vi "Response Check.vi"(6 "Source (\"\")":string, 8 "error in (no error)":errorcluster, 9 "Message In (\"\")":string, 11 "VISA resource name":refnum<visa-resource-name>) -> (0 "error out":errorcluster, 1 "Internal Error Number":i32 max=999 step=1, 2 "Response Type":i32(ring) items=["Affirmative", "Single Negative", "Multiple Negative", "ASCII", "Binary", "End"], 3 "VISA resource name out":refnum<visa-resource-name>, 4 "Internal Error String":string)   [LabVIEW 2020, in "Yokogawa GX Series.lvlib"]
doc: "This VI checks the message.\nThen this returns Internal Error Type.\nIf the message is an error message, this sets \"command are not processed succesfully\" to error out."
uses:
  <instrlib>/Yokogawa GX Series/Yokogawa GX Series.lvlib
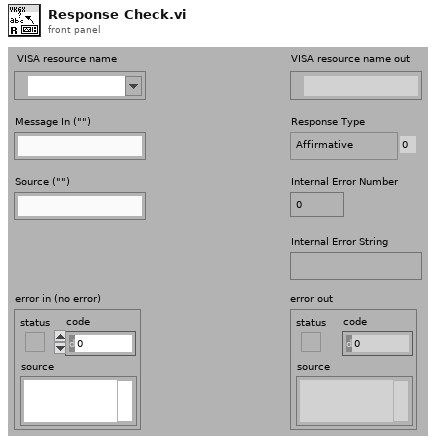
[diagram p1: front panel]
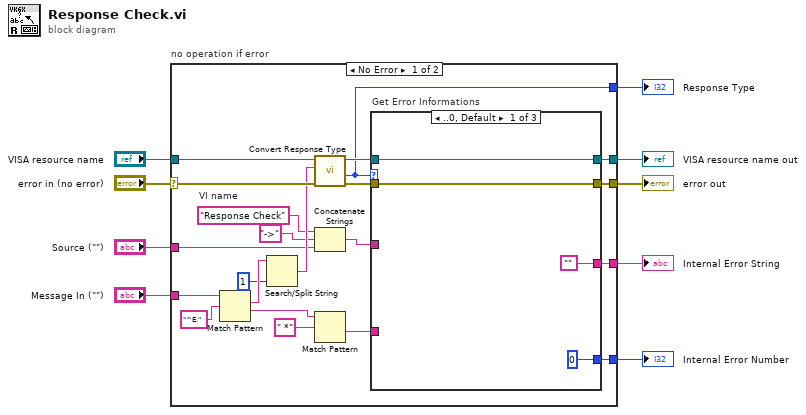
[diagram p0: block diagram]
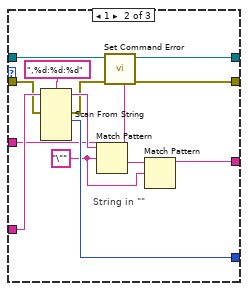
[diagram p2: hidden frame]
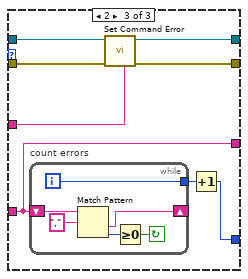
[diagram p3: hidden frame]
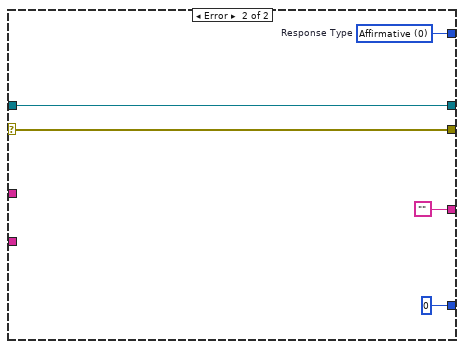
[diagram p4: hidden frame]
diagram:
  n1 = case "no operation if error" shown="No Error" "error in (no error)" {
    selector: "error in (no error)" -> [w15 w65]
    tunnel: [w28 w65] -> w5
    tunnel: "Message In (\"\")" -> [w27 _]
    tunnel: [w30 0] -> w3
    tunnel: [w29 ""] -> w4
    tunnel: [w18 w63] -> w7
    tunnel: "VISA resource name" -> [w16 w66]
    tunnel: [w20 w66] -> w6
    tunnel: "Source (\"\")" -> [w11 _]
    frame No Error {
      w10 = "Response Check"  # VI name
      n2 = Match Pattern(string=w27, regular expression="^E.") -> (match substring=w23:string, after substring=w21:string)  [unwired: 3 out]
      n3 = Search/Split String(string=w23, offset (0)=1) -> (match + rest of string=w14:string)  [unwired: 3 out]
      n4 = call <instrlib>:"Convert Response Type.vi"("error in (no error)"=w15, "Response Type String (\"\")"=w14, "VISA resource name"=w16) -> ("error out"=w17:errorcluster, "Response Type"=w18:i32, "VISA resource name out"=w19:refnum<visa-resource-name>)  [unwired: 6 out]
      n5 = Concatenate Strings(w10, "->", w11) -> (w13:string)
      n6 = Match Pattern(string=w21, regular expression=" *") -> (after substring=w24:string)  [unwired: 4 out]
      n7 = case "Get Error Informations" shown="..0, Default" w18 {
        tunnel: [0 w46 w54] -> w30
        tunnel: ["" w43 w53] -> w29
        tunnel: w17 -> [w34 w41 w49]
        tunnel: [w34 w38 w51] -> w28
        tunnel: w24 -> [_ w42 w53]
        tunnel: w19 -> [w33 w35 w48]
        tunnel: [w33 w39 w52] -> w20
        tunnel: w13 -> [_ w36 w50]
        frame ..0, Default {
        }
        frame 1 {
          w40 = "\""
          # "String in \"\""
          n8 = Scan From String(format string=",%d:%d:%d", input string=w42, error in=w41) -> (remaining string=w45:string, error out=w37:errorcluster, output 1=w46:i32)  [unwired: 1 in, 6 out]
          n9 = Match Pattern(string=w45, regular expression=w40) -> (after substring=w44:string)  [unwired: 4 out]
          n10 = call <instrlib>:"Set Command Error.vi"("Source (\"\")"=w36, "error in (no error)"=w37, "VISA resource name"=w35) -> ("error out"=w38:errorcluster, "VISA resource name out"=w39:refnum<visa-resource-name>)  [unwired: 7 out]
          n11 = Match Pattern(string=w44, regular expression=w40) -> (before substring=w43:string)  [unwired: 4 out]
        }
        frame 2 {
          n12 = while "count errors" {
            tunnel: [w56] -> w55
            shift-left: w53 -> [w61]
            shift-right: [w59] -> _
            i -> [w56]
            stop <- w57 continue-if-true
            n13 = Match Pattern(string=w61, regular expression=",") -> (after substring=w59:string, offset past match=w58:i32)  [unwired: 3 out]
            n14 = Greater Or Equal To 0?(x=w58) -> (x >= 0?=w57:bool)
          }
          n15 = call <instrlib>:"Set Command Error.vi"("Source (\"\")"=w50, "error in (no error)"=w49, "VISA resource name"=w48) -> ("error out"=w51:errorcluster, "VISA resource name out"=w52:refnum<visa-resource-name>)  [unwired: 7 out]
          n16 = Increment(x=w55) -> (x+1=w54:i32)
        }
      }
    }
    frame Error {
      w63 = 0 items=["Affirmative", "Single Negative", "Multiple Negative", "ASCII", "Binary", "End"]  # Response Type
    }
  }
  "error out" <- w5
  "VISA resource name out" <- w6
  "Internal Error Number" <- w3
  "Internal Error String" <- w4
  "Response Type" <- w7
